vi "SwerveDriveNormalize.vi"(1 "Motor Speed In":dbl[](array[numeric])) -> (0 "Motor Speed Out":dbl[](array[numeric]))   [LabVIEW 2019, in "Swerve Drive.lvlib"]
uses:
  Swerve Drive.lvlib
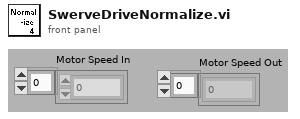
[diagram p1: front panel]
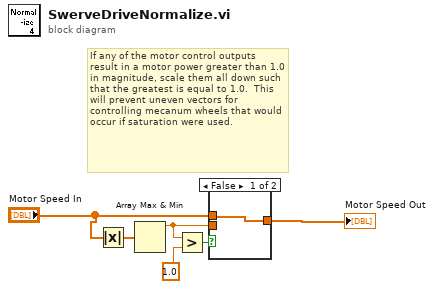
[diagram p0: block diagram]
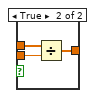
[diagram p2: hidden frame]
diagram:
  # "If any of the motor control outputs result in a motor power greater than 1.0 in magnitude, scale them all down such that the greatest is equal to 1.0.  This will prevent uneven vectors for controlling mecanum wheels that would occur if saturation were used."
  n1 = Absolute Value(x="Motor Speed In") -> (abs(x)=w6:dbl[])
  n2 = Array Max & Min(array=w6) -> (max value=w4:dbl)  [unwired: 3 out]
  n3 = Greater?(x=w4, y=1.0) -> (0:w5:bool)
  n4 = case shown="False" w5 {
    tunnel: w4 -> [_ w10]
    tunnel: [w7 w9] -> w1
    tunnel: "Motor Speed In" -> [w7 w8]
    frame False {
    }
    frame True {
      n5 = Divide(x=w8, y=w10) -> (x/y=w9:dbl[])
    }
  }
  "Motor Speed Out" <- w1
